vi "Launch Panel Thread.vi"(8 "error in (no error)":errorcluster, 10 "Front Panel Window:Title(\"\")":string, 11 "Panel Manager Controller.lvclass":refnum<class "Panel Manager Controller.lvclass">) -> (0 "error out":errorcluster, 3 "Panel Manager Controller.lvclass out":refnum<class "Panel Manager Controller.lvclass">)   [LabVIEW 2015, in "Panel Manager Controller.lvclass"]
uses:
  Panel Manager Controller.lvclass
  Panel Control_Ref/Panel Controller.lvclass
  <vilib>/ActorFramework/Actor/Actor.lvclass/Actor.ctl
  <vilib>/ActorFramework/Message Enqueuer/Message Enqueuer.lvclass/Message Enqueuer.ctl
  Panel Manager Controller.lvclass/Panel Manager Controller.ctl
  Panel View/Panel View.lvclass/Panel View.ctl
  <vilib>/ActorFramework/Message Enqueuer/Init from Existing Queue.vi
  <vilib>/ActorFramework/Message Enqueuer/Message Enqueuer.lvclass
  Panel View/Panel View.lvclass
  <vilib>/ActorFramework/Actor/Actor.lvclass
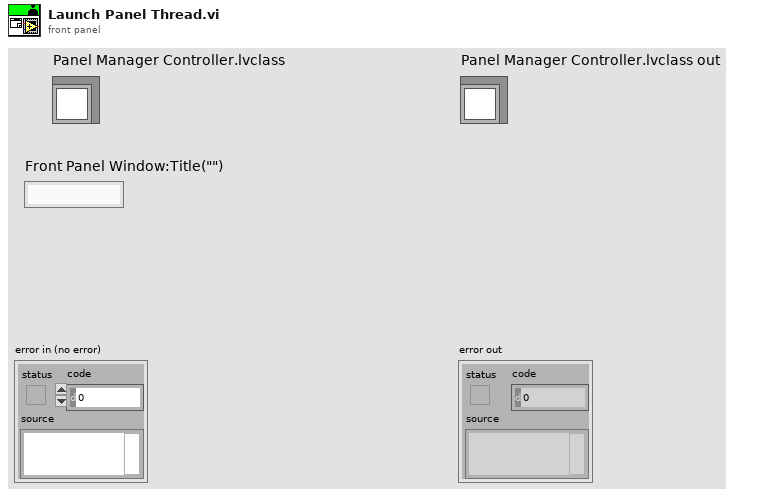
[diagram p1: front panel]
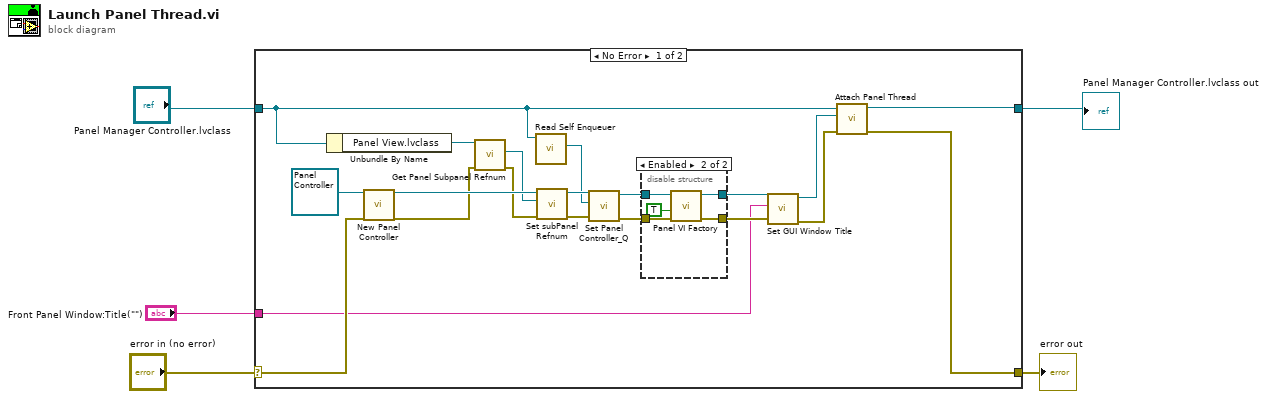
[diagram p0: block diagram]
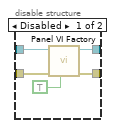
[diagram p2: hidden frame]
diagram:
  n1 = case shown="No Error" "error in (no error)" {
    selector: "error in (no error)" -> [w25 w37]
    tunnel: [w23 w37] -> w4
    tunnel: [w24 w36] -> w1
    tunnel: "Panel Manager Controller.lvclass" -> [w16 w36]
    tunnel: "Front Panel Window:Title(\"\")" -> [w6 _]
    frame No Error {
      n2 = Unbundle By Name(w16) -> ("Panel View.lvclass"=w20:refnum<class "Panel View.lvclass">)
      n3 = call "New Panel Controller.vi"("reference in"=refnum<class "Panel Controller.lvclass"> refnum, "error in (no error)"=w25) -> ("reference out"=w22:refnum<class "Panel Controller.lvclass">, "error out"=w19:errorcluster)  [unwired: 16 in]
      n4 = call "Get Panel Subpanel Refnum.vi"("error in (no error)"=w19, "Panel View in"=w20) -> ("error out"=w18:errorcluster, "Panel Subpanel Refnum"=w17:refnum<vi>)  [unwired: 7 in, 1 out]
      n5 = call <vilib>:"Read Self Enqueuer.vi"("Actor"=w16) -> ("Self Enqueuer"=w11:refnum<class "Message Enqueuer.lvclass">)  [unwired: 10 in]
      n6 = call "Set subPanel Refnum.vi"("error in (no error)"=w18, "Sub Panel Ref"=w17, "Panel Control_Ref in"=w22) -> ("error out"=w14:errorcluster, "Panel Control_Ref out"=w15:refnum<class "Panel Controller.lvclass">)  [unwired: 7 in]
      n7 = call "Set Panel Controller_Q.vi"("error in (no error)"=w14, "Panel Controller_Q"=w11, "Panel Control_Ref in"=w15) -> ("error out"=w12:errorcluster, "Panel Control_Ref out"=w13:refnum<class "Panel Controller.lvclass">)  [unwired: 7 in]
      n8 = disable-structure shown="Enabled" {
        disable-tunnel: [w30 w32] -> w9
        disable-tunnel: [w29 w34] -> w10
        disable-tunnel: w13 -> [w27 w35]
        disable-tunnel: w12 -> [w26 w33]
        frame Disabled {
          n9 = call "Panel VI Factory.vi"("SubPanel?(False)"=TRUE, "error in (no error)"=w26, "Panel Control_Ref in"=w27) -> ("error out"=w30:errorcluster, "Panel Control_Ref out"=w29:refnum<class "Panel Controller.lvclass">)  [unwired: 7 in]
        }
        frame Enabled {
          n10 = call "Panel VI Factory.vi"("error in (no error)"=w33, "Open?(True)"=TRUE, "Panel Control_Ref in"=w35) -> ("error out"=w32:errorcluster, "Panel Control_Ref out"=w34:refnum<class "Panel Controller.lvclass">)  [unwired: 7 in]
        }
      }
      n11 = call "Set GUI Window Title.vi"("error in (no error)"=w9, "Front Panel Window:Title"=w6, "Panel Control_Ref in"=w10) -> ("error out"=w7:errorcluster, "Panel Control_Ref out"=w8:refnum<class "Panel Controller.lvclass">)  [unwired: 7 in]
      n12 = call "Attach Panel Thread.vi"("error in (no error)"=w7, "Panel Thread"=w8, "Panel Manager Controller.lvclass"=w16) -> ("error out"=w23:errorcluster, "Panel Manager Controller.lvclass out"=w24:refnum<class "Panel Manager Controller.lvclass">)  [unwired: 7 in]
    }
    frame Error {
    }
  }
  "error out" <- w4
  "Panel Manager Controller.lvclass out" <- w1
